vi "数据查询_报警信息.vi"() -> ()   [LabVIEW 2016]
uses:
  <vilib>/Utility/miscctls.llb/LVPointTypeDef.ctl
  <vilib>/Utility/miscctls.llb/LVRowAndColumnUnsignedTypeDef.ctl
  <userlib>/_OpenG.lib/array/array.llb/Sort 2D Array (String)__ogtk.vi
panel:
  in  "下拉列表":string(xcontrol)
  in  "导出":bool
  in  "查询":bool
  in  "结束日期":string="2050/01/01"
  in  "起始日期":string="2010/01/01"
  out "数据表":string[][](table)
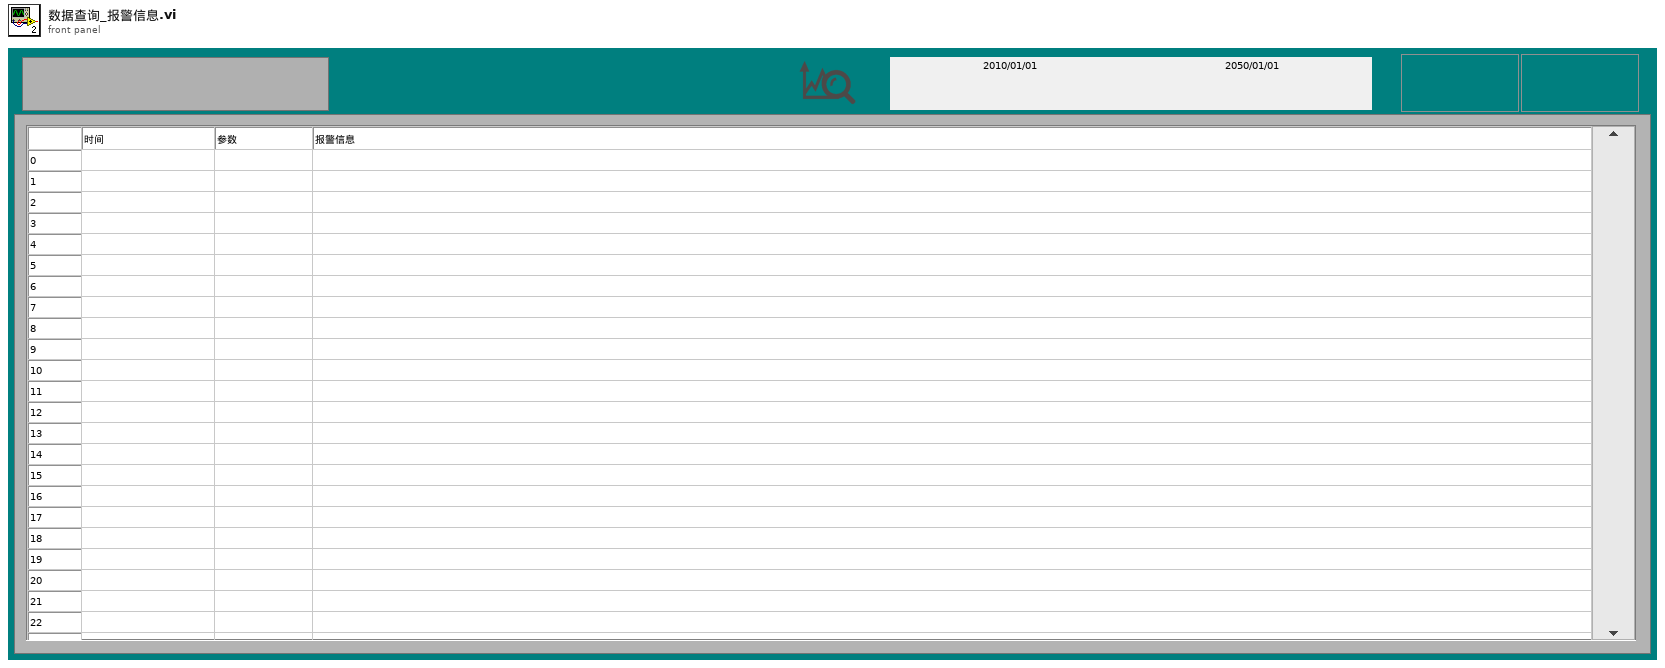
[diagram p1: front panel]
types:
  T1 = enum8{"Enabled", "Disabled", "Disabled and Grayed Out"}
  T2 = typedef "LVRowAndColumnUnsignedTypeDef.ctl" = cluster{"Row":u32, "Column":u32}
  T3 = typedef "LVPointTypeDef.ctl" = cluster{"Horizontal":i16, "Vertical":i16}
  T4 = typedef "LVDateTimeRec.ctl" = cluster{"秒数的小数部分":dbl, "秒":i32, "分":i32, "时":i32, "日":i32, "月":i32, "年":i32, "天数（周）":i32, "天数（年）":i32, "DST":i32}
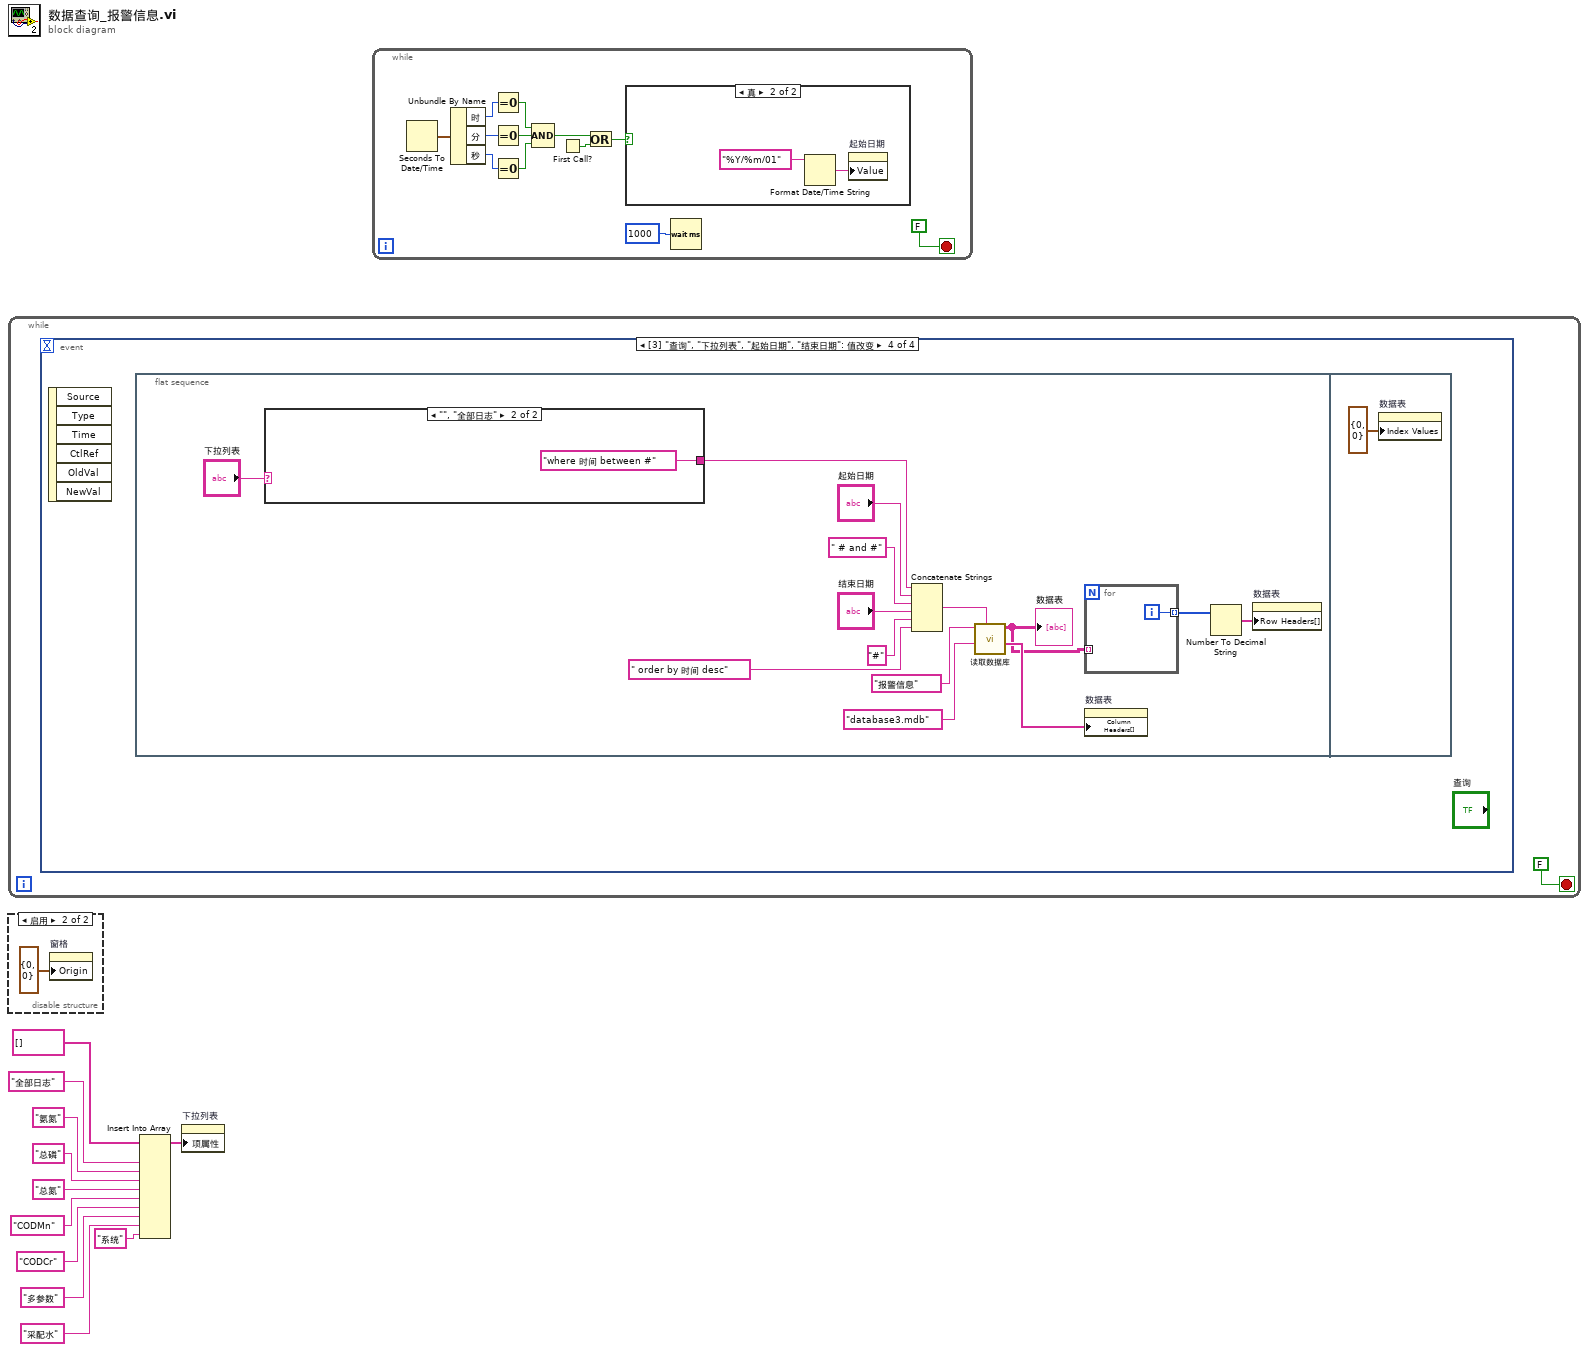
[diagram p0: block diagram]
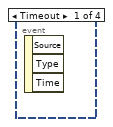
[diagram p3: hidden frame]
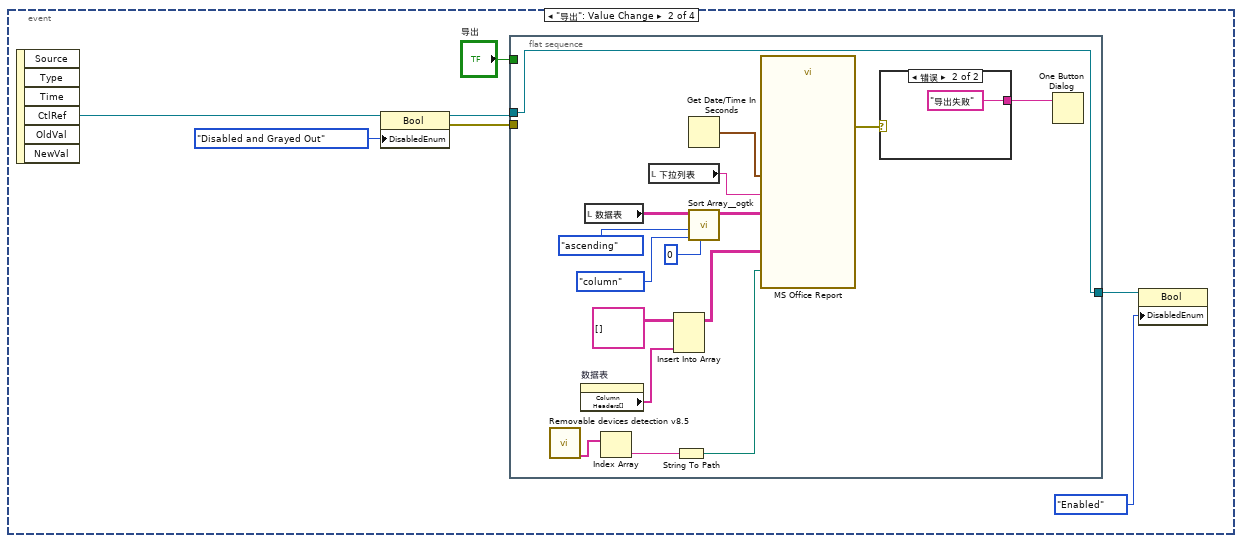
[diagram p4: hidden frame]
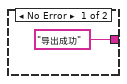
[diagram p5: hidden frame]
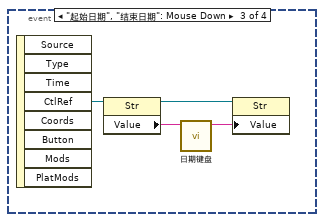
[diagram p6: hidden frame]
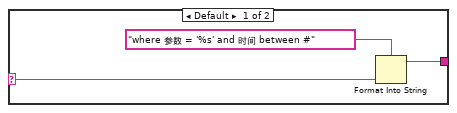
[diagram p7: hidden frame]
diagram:
  n1 = while {
    stop <- FALSE stop-if-true
    n2 = event shown="[3] \"查询\", \"下拉列表\", \"起始日期\", \"结束日期\": 值改变" {
      selector: _ -> [_ _ _ _]
      dyn-events: _ -> [_ _ _ _]
      timeout: _ -> [_ _ _ _]
      event Timeout {
        n3 = event-data() -> ()  [unwired: 1 in, 3 out]
      }
      event "导出": Value Change {
        n4 = event-data() -> ("CtlRef"=w13:refnum<vi>)  [unwired: 1 in, 5 out]
        n5 = property class="Bool"(reference=w13, "DisabledEnum"=T1."Disabled and Grayed Out" ("禁用")) -> (reference out=w17:refnum<vi>, error out=w18:errorcluster)  [unwired: 1 in]
        n6 = flat-sequence {
          tunnel: w18 -> [_]
          tunnel: [w28] -> w16
          tunnel: w17 -> [w28]
          tunnel: "导出" -> [_]
          frame #0 {
            n7 = call "Removable devices detection v8.5.vi"() -> ("Removable"=w25:string[])  [unwired: 4 out]
            n8 = property on="数据表" class="Tbl (严格)"() -> ("Column Headers[]"=w21:string[])  [unwired: 2 in, 2 out]
            n9 = local read "数据表"() -> (w34:string[][])
            n10 = Index Array(array=w25) -> (element=w24:string)  [unwired: 1 in]
            n11 = local read "下拉列表"() -> (w29:string)
            n12 = Insert Into Array(array=string[][] [], new element=w21) -> (w20:string[][])  [unwired: 2 in]
            n13 = String To Path(string=w24) -> (path=w23:path)
            n14 = Get Date/Time In Seconds() -> (seconds since 1Jan1904=w35:timestamp)
            n15 = call-poly <userlib>:"Sort Array__ogtk.vi"("Column/Row to Sort By"=u32 0, "Sort By in"=enum16{"row", "column"}."column", "Order"=enum16{"ascending", "descending"}."ascending", "Array in"=w34) -> ("Sorted Array out"=w33:string[][])  [unwired: 4 in, 3 out]
            n16 = call "MS Office Report"("Path to Save Report"=w23, "导出日期"=w35, "监测参数"=w29, "数据输入"=w33, "字段定义"=w20) -> ("error out"=w27:errorcluster)  [unwired: 21 in, 1 out]
            n17 = case shown="错误" w27 {
              tunnel: ["导出成功" ("消息") "导出失败" ("消息")] -> w26
              frame No Error {
              }
              frame Error {
              }
            }
            n18 = One Button Dialog(message=w26) -> ()  [unwired: 1 in, 1 out]
          }
        }
        n19 = property class="Bool"(reference=w16, "DisabledEnum"=T1."Enabled" ("禁用")) -> ()  [unwired: 1 in, 2 out]
      }
      event "起始日期", "结束日期": Mouse Down {
        n20 = event-data() -> ("CtlRef"=w41:refnum<vi>)  [unwired: 1 in, 7 out]
        n21 = property class="Str"(reference=w41) -> (reference out=w39:refnum<vi>, "Value"=w40:string)  [unwired: 1 in, 1 out]
        n22 = call "日期键盘.vi"("原值"=w40) -> ("x+y"=w38:string)  [unwired: 10 in]
        n23 = property class="Str"(reference=w39, "Value"=w38) -> ()  [unwired: 1 in, 2 out]
      }
      event "查询", "下拉列表", "起始日期", "结束日期": Value Change {
        n24 = event-data() -> ()  [unwired: 1 in, 6 out]
        n25 = flat-sequence {
          frame #0 {
            n26 = case shown="\"\", \"全部日志\"" "下拉列表" {
              selector: "下拉列表" -> [w56 _]
              tunnel: [w58 "where 时间 between #" ("condition")] -> w43
              frame Default {
                n27 = Format Into String(format string="where 参数 = '%s' and 时间 between #" ("condition"), w56) -> (resulting string=w58:string)  [unwired: 2 in, 1 out]
              }
              frame "", "全部日志" {
              }
            }
            n28 = Concatenate Strings(w43, "起始日期", " # and #" ("condition"), "结束日期", "#" ("condition"), " order by 时间 desc" ("字符串")) -> (w54:string)
            n29 = call "读取数据库.vi"("condition"=w54, "database"="database3.mdb", "组合框"="报警信息") -> ("columns"=w50:string[], "表格"=w48:string[][])  [unwired: 5 in, 2 out]
            "数据表" <- w48
            n30 = for {
              tunnel: w48 -> [_] mode=indexing
              tunnel: [w60] -> w47 mode=indexing
              i -> [w60]
            }
            n31 = property on="数据表" class="Tbl (严格)"("Column Headers[]"=w50) -> ()  [unwired: 2 in, 2 out]
            n32 = Number To Decimal String(number=w47) -> (decimal integer string=w46:string[])  [unwired: 1 in]
            n33 = property on="数据表" class="Tbl (严格)"("Row Headers[]"=w46) -> ()  [unwired: 2 in, 2 out]
          }
          frame #1 {
            n34 = property on="数据表" class="Tbl (严格)"("Index Values"=T2 {"Row"=0, "Column"=0} ("索引值")) -> ()  [unwired: 2 in, 2 out]
          }
        }
      }
    }
  }
  n35 = disable-structure shown="启用" {
    frame Disabled {
    }
    frame Enabled {
      n36 = property on="窗格" class="Pane"("Origin"=T3 {"Horizontal"=0, "Vertical"=0} ("原点")) -> ()  [unwired: 2 in, 2 out]
    }
  }
  n37 = Insert Into Array(array=string[] [], new element #1="全部日志" ("新元素/子数组"), new element #2="氨氮" ("新元素/子数组"), new element #3="总磷" ("新元素/子数组"), new element #4="总氮" ("新元素/子数组"), new element #5="CODMn" ("新元素/子数组"), new element #6="CODCr" ("新元素/子数组"), new element #7="多参数" ("新元素/子数组"), new element #8="采配水" ("新元素/子数组"), new element #9="系统" ("新元素/子数组")) -> (w1:string[])  [unwired: 1 in]
  n38 = property on="下拉列表" class="下拉列表 (严格)"("项属性"=w1) -> ()  [unwired: 2 in, 2 out]
  n39 = while {
    stop <- FALSE stop-if-true
    n40 = Seconds To Date/Time() -> (date time rec=w74:T4)  [unwired: 2 in]
    n41 = Unbundle By Name(w74) -> ("时"=w73:i32, "分"=w72:i32, "秒"=w71:i32)
    n42 = Equal To 0?(x=w73) -> (x = 0?=w70:bool)
    n43 = Equal To 0?(x=w72) -> (x = 0?=w69:bool)
    n44 = Equal To 0?(x=w71) -> (x = 0?=w68:bool)
    n45 = Compound Arithmetic op=AND ("复合运算")(w70, w69, w68) -> (w65:bool)
    n46 = First Call?() -> (First Call?: T/F=w63:bool)
    n47 = Or(x=w65, y=w63) -> (x .or. y?=w64:bool)
    n48 = case shown="真" w64 {
      frame False {
      }
      frame True {
        n49 = Format Date/Time String(time format string (%c)="%Y/%m/01" ("时间格式字符串(%c)")) -> (date/time string=w75:string)  [unwired: 2 in]
        n50 = property on="起始日期" class="Str"("Value"=w75) -> ()  [unwired: 2 in, 2 out]
      }
    }
    n51 = Wait (ms)(milliseconds to wait=u32 1000 ("等待时间（毫秒）")) -> ()  [unwired: 1 out]
  }
